vi "SOAP解析.vi"(7 "DATA":string, 8 "错误输入（无错误）":errorcluster, 10 "Headers":string[][](array[string])=[["Content-Type", "text/xml;charset=UTF-8"], ["SOAPAction", "\"http://tempuri.org/ICalbProductParaColloctUniversalWcf/productParaColloctUniversal\""], ["Connection", "Keep-Alive"], ["User-Agent", "Apache-HttpClient/4.1.1 (java 1.5)"]], 11 "URL":string) -> (0 "错误输出":errorcluster, 1 "body":string, 2 "headers":string caption="头部")   [LabVIEW 2015]
uses:
  <vilib>/httpClient/POSTBuffer.vi
  <vilib>/httpClient/LabVIEWHTTPClient.lvlib
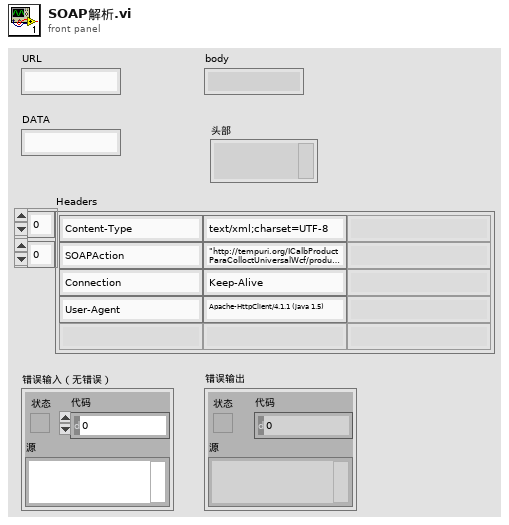
[diagram p1: front panel]
types:
  T1 = typedef "LabVIEWHTTPClient.lvlib/ClientHandle.ctl" = refnum<k1>
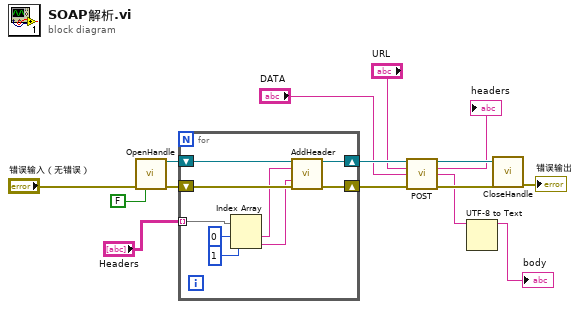
[diagram p0: block diagram]
diagram:
  n1 = call <vilib>:"OpenHandle.vi"("error in (no error)"="错误输入（无错误）", "verify server(true)"=FALSE) -> ("client handle out"=w12:T1, "error out"=w13:errorcluster)  [unwired: 12 in]
  n2 = for {
    shift-right: [w19] -> w11
    shift-left: w12 -> [w20]
    shift-right: [w21] -> w14
    shift-left: w13 -> [w22]
    tunnel: "Headers" -> [w16] mode=indexing
    n3 = Index Array(array=w16, index #1=0 ("index"), index #2=1 ("index")) -> (element #1=w18:string, element #2=w17:string)
    n4 = call <vilib>:"AddHeader.vi"("client handle"=w20, "header"=w18, "value"=w17, "error in (no error)"=w22) -> ("client handle out"=w19:T1, "error out"=w21:errorcluster)  [unwired: 10 in]
  }
  n5 = call-poly <vilib>:"POST.vi"("client handle"=w11, "url"="URL", "buffer"="DATA", "error in (no error)"=w14) -> ("client handle out"=w7:T1, "headers"=→"headers":string, "body"=w2:string, "error out"=w6:errorcluster)  [unwired: 8 in]
  n6 = UTF-8 to Text(11:w2) -> (3:→"body":string)  [unwired: 2 in, 1 out]
  n7 = call <vilib>:"CloseHandle.vi"("client handle"=w7, "error in (no error)"=w6) -> ("error out"=→"错误输出":errorcluster)  [unwired: 13 in]
